vi "Query - Tree Info Input_SubVIs-某型振动实验台测试系统.vi"(7 "Tree引用句柄":refnum<vi>, 8 "错误输入（无错误）":errorcluster, 10 "units":string[](array[string]), 11 "Vibration Channel Name Output":string[](array[string])) -> (0 "错误输出":errorcluster)   [LabVIEW 2011]
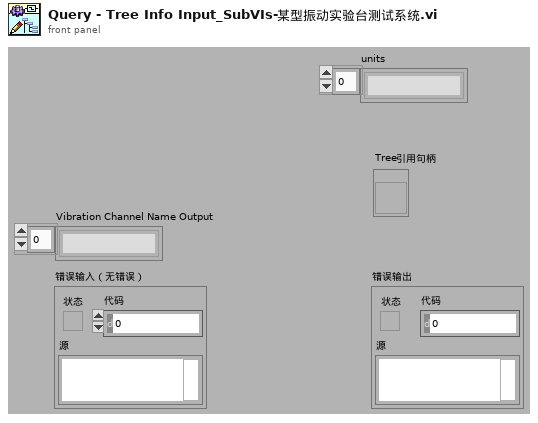
[diagram p1: front panel]
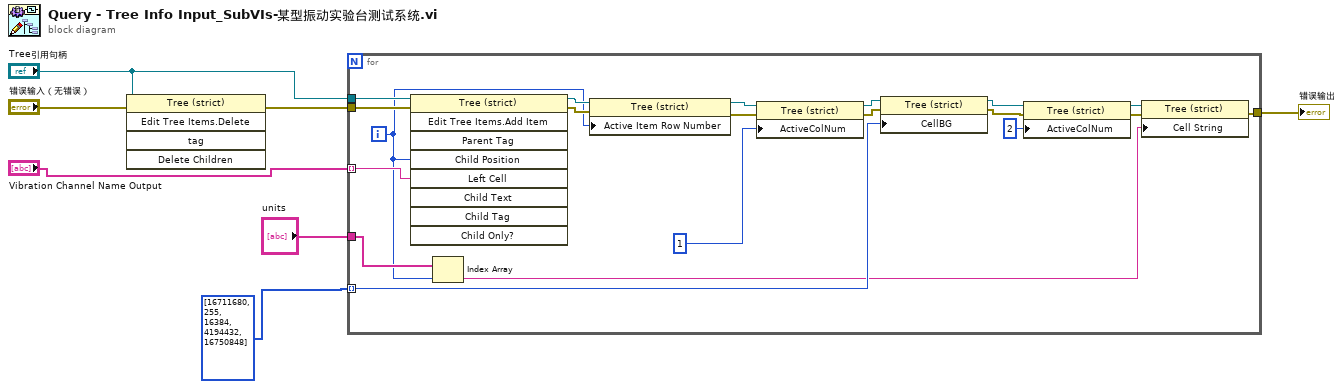
[diagram p0: block diagram]
diagram:
  n1 = invoke on="调用节点" class="Tree (strict)" method="Edit Tree Items.Delete"(reference="Tree引用句柄", error in="错误输入（无错误）") -> (error out=w7:errorcluster)  [unwired: 3 in, 4 out]
  n2 = for {
    tunnel: w7 -> [w27]
    tunnel: "Tree引用句柄" -> [w26]
    tunnel: "Vibration Channel Name Output" -> [w25] mode=indexing
    tunnel: u32[] [16711680, 255, 16384, 4194432, 16750848] -> [w21] mode=indexing
    tunnel: "units" -> [w10]
    tunnel: [w12] -> w1
    i -> [w8]
    n3 = invoke on="调用节点" class="Tree (strict)" method="Edit Tree Items.Add Item"(reference=w26, error in=w27, "Child Position"=w8, "Left Cell"=w25) -> (reference out=w20:refnum<vi>, error out=w18:errorcluster)  [unwired: 5 in, 7 out]
    n4 = Index Array(array=w10, index=w8) -> (element=w9:string)
    n5 = property class="Tree (strict)"(reference=w20, error in=w18, "Active Item Row Number"=w8) -> (reference out=w19:refnum<vi>, error out=w17:errorcluster)
    n6 = property class="Tree (strict)"(reference=w19, error in=w17, "ActiveColNum"=1 ("活动单元格:活动列数")) -> (reference out=w23:refnum<vi>, error out=w22:errorcluster)
    n7 = property class="Tree (strict)"(reference=w23, error in=w22, "CellBG"=w21) -> (reference out=w16:refnum<vi>, error out=w11:errorcluster)
    n8 = property class="Tree (strict)"(reference=w16, error in=w11, "ActiveColNum"=2 ("活动单元格:活动列数")) -> (reference out=w14:refnum<vi>, error out=w13:errorcluster)
    n9 = property class="Tree (strict)"(reference=w14, error in=w13, "Cell String"=w9) -> (error out=w12:errorcluster)  [unwired: 1 out]
  }
  "错误输出" <- w1
